vi "regTel.vi"(8 "error in (no error)":errorcluster, 10 "telReg":string[][](array[string]), 11 "tcpServer in":refnum<class "TcpServer.lvclass">) -> (0 "error out":errorcluster, 3 "tcpServer out":refnum<class "TcpServer.lvclass">)   [LabVIEW 2018, in "TcpServer.lvclass"]
doc: "Inform the TCP Server which telemetry is registered and allowed to be used by LabVIEW Component. For instance,\n\n| compName | telName |\n| ---------------- | ------------- |\n| Dome | position |"
uses:
  TcpServer.lvclass
  TcpServer.lvclass/TcpServer.ctl
  TcpServerBase/TcpServerBase.lvclass/TcpServerBase.ctl
  TcpServerTel/TcpServerTel.lvclass
  home/pcortes/github/ts_labview_tcp_json/src/TcpServerBase/TcpServerBase.lvclass
  TcpServerBase/TcpServerBase.lvclass
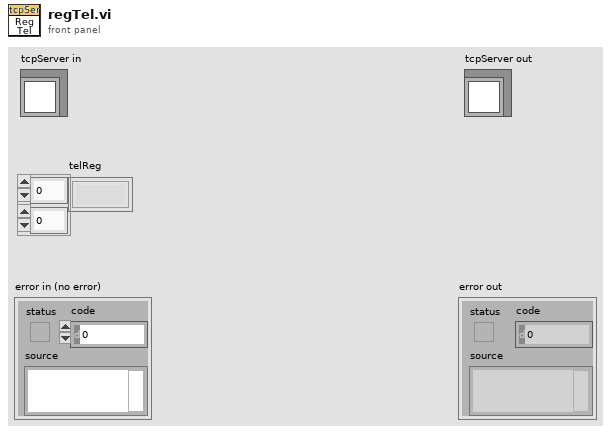
[diagram p1: front panel]
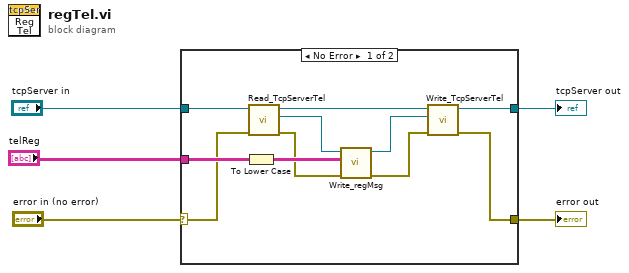
[diagram p0: block diagram]
diagram:
  n1 = case shown="No Error" "error in (no error)" {
    selector: "error in (no error)" -> [w13 w18]
    tunnel: [w11 w18] -> w4
    tunnel: [w12 w17] -> w2
    tunnel: "tcpServer in" -> [w15 w17]
    tunnel: "telReg" -> [w16 _]
    frame No Error {
      n2 = To Lower Case(string=w16) -> (all lower case string=w10:string[][])
      n3 = call "Read_TcpServerTel.vi"("error in (no error)"=w13, "TcpServer in"=w15) -> ("error out"=w7:errorcluster, "TcpServerTel.lvclass"=w9:refnum<class "TcpServerTel.lvclass">, "TcpServer out"=w14:refnum<class "TcpServer.lvclass">)  [unwired: 7 in]
      n4 = call "Write_regMsg.vi"("error in (no error)"=w7, "regMsg"=w10, "TcpServerBase in"=w9) -> ("error out"=w6:errorcluster, "TcpServerBase out"=w8:refnum<class "TcpServerTel.lvclass">)  [unwired: 7 in]
      n5 = call "Write_TcpServerTel.vi"("error in (no error)"=w6, "TcpServerTel.lvclass"=w8, "TcpServer in"=w14) -> ("error out"=w11:errorcluster, "TcpServer out"=w12:refnum<class "TcpServer.lvclass">)  [unwired: 7 in]
    }
    frame Error {
    }
  }
  "error out" <- w4
  "tcpServer out" <- w2
